vi "OffDelay_Example.vi"() -> ()   [LabVIEW 2019]
uses:
  <vilib>/Rock Robotics/WPI/ThirdParty/JAS_Junk/TrajLib/Timer_New.vi
  <vilib>/Utility/semaphor.llb/Obtain Semaphore Reference.vi
  <vilib>/Rock Robotics/WPI/ThirdParty/JAS_Junk/TrajLib/Timer_Reset.vi
  <vilib>/Rock Robotics/WPI/ThirdParty/JAS_Junk/TrajLib/Timer_Start.vi
  <vilib>/Rock Robotics/WPI/ThirdParty/JAS_Junk/TrajLib/Timer_HasPeriodPassedOnce.vi
  <vilib>/Rock Robotics/WPI/ThirdParty/JAS_Junk/TrajLib/Timer_Stop.vi
  <vilib>/Rock Robotics/WPI/ThirdParty/JAS_Junk/TrajLib/Trajectory_Library.lvlib
panel:
  out "OFF DELAY":cluster{i16, i16}(graph)
  out "Remaining Time\nSeconds":dbl format="%14.2f"
  in  "Delay\nSeconds":dbl=10.0
  out "Ouptut":bool
  in  "Input":bool
  # "OFF DELAY EXAMPLE"
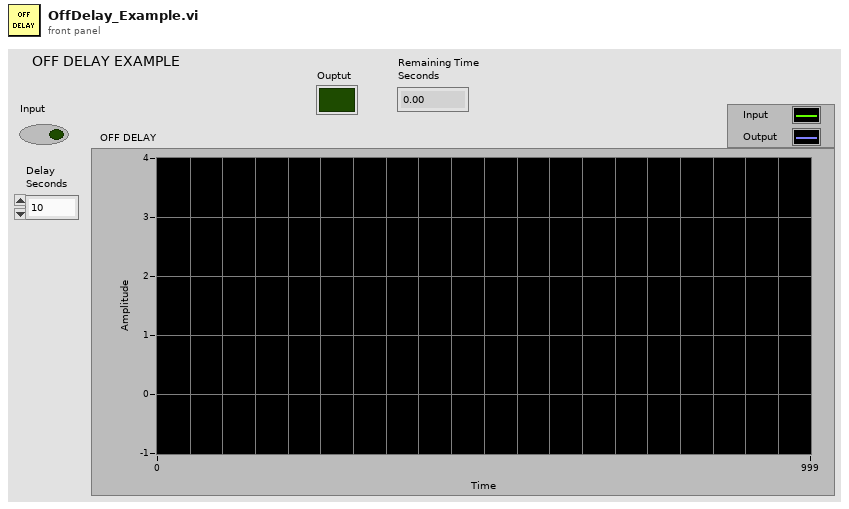
[diagram p1: front panel]
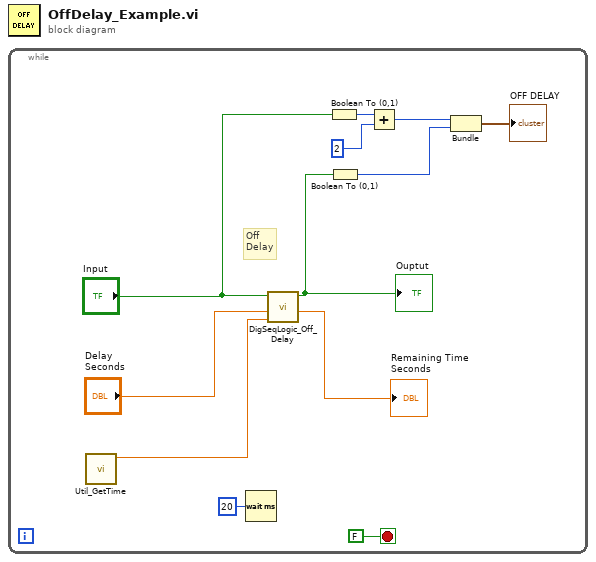
[diagram p0: block diagram]
diagram:
  n1 = while {
    stop <- FALSE stop-if-true
    # "Off\nDelay"
    n2 = call <vilib>:"Util_GetTime.vi"() -> ("FPGA_Time_Seconds"=w8:dbl)  [unwired: 10 in, 1 out]
    n3 = Wait (ms)(milliseconds to wait=u32 20) -> ()  [unwired: 1 out]
    n4 = call <vilib>:"DigSeqLogic_Off_Delay.vi"("Time"=w8, "Delay"="Delay\nSeconds", "Input"="Input") -> ("Remain"=→"Remaining Time\nSeconds":dbl, "Output"=w6:bool)  [unwired: 7 in]
    "Ouptut" <- w6
    n5 = Boolean To (0,1)(Boolean="Input") -> (0, 1=w3:i16)
    n6 = Boolean To (0,1)(Boolean=w6) -> (0, 1=w1:i16)
    n7 = Add(x=w3, y=i16 2) -> (x+y=w2:i16)
    n8 = Bundle(w2, w1) -> (→"OFF DELAY":cluster{i16, i16})  [unwired: 1 in]
  }
